vi "Text to Timestamp.vi"(8 "error in (no error)":errorcluster, 9 "initial scan location":u32, 11 "Text Timestamp":string) -> (0 "error out":errorcluster, 1 "Offset Past Timestamp":u32, 2 "Local Time Offset (NaN if unspecified)":dbl, 3 "Time Stamp":timestamp format="%^<%H:%M:%S%6u\n%Y/%m/%d>T UTC")   [LabVIEW 2024, in "JDP Timestamp.lvlib"]
doc: "Supporting RFC3339, a subset of ISO8601, plus some other formats \nRFC3339--> https://tools.ietf.org/html/rfc3339 \n Examples:\n \"2020-06-25T08:50:15.123Z\"\n \"2020-06-25T09:50:15.123+01:00\"\n\nSQLite Time Functions --> https://www.sqlite.org/lang_datefunc.html\n Examples:\n \"2020-06-25 08:50:15\" --> datetime() function\n\nAlso accepts reduced formats omitting some of the separators, or replacing them with spaces:\n \"2020 06 25 085015Z\"\n\nTo support older versions of Windows Powershell (ConvertTo-Json commandlet), also supports milliseconds since the Unix Epoch, in /Date(nnn)/ format:\n \"/Date(1608992240123)/\""
uses:
  JDP Timestamp.lvlib
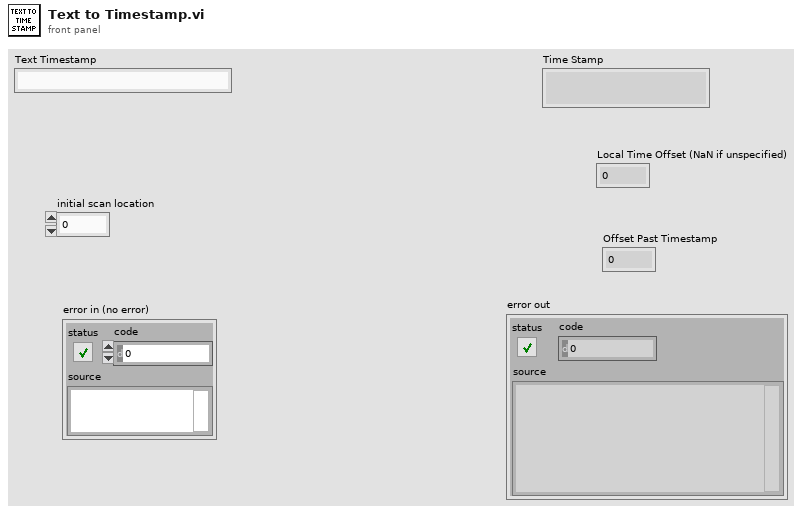
[diagram p1: front panel]
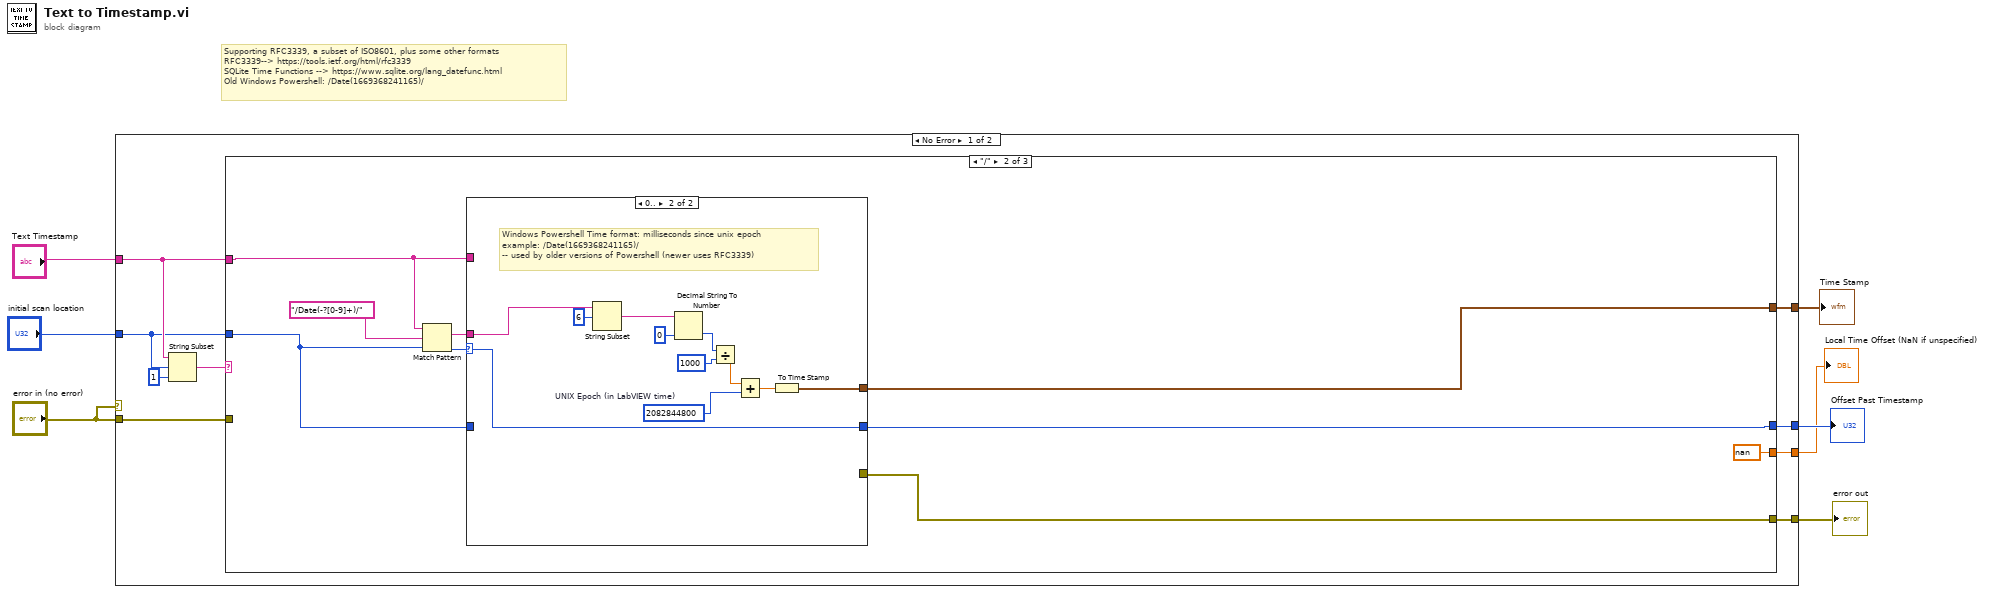
[diagram p0: block diagram]
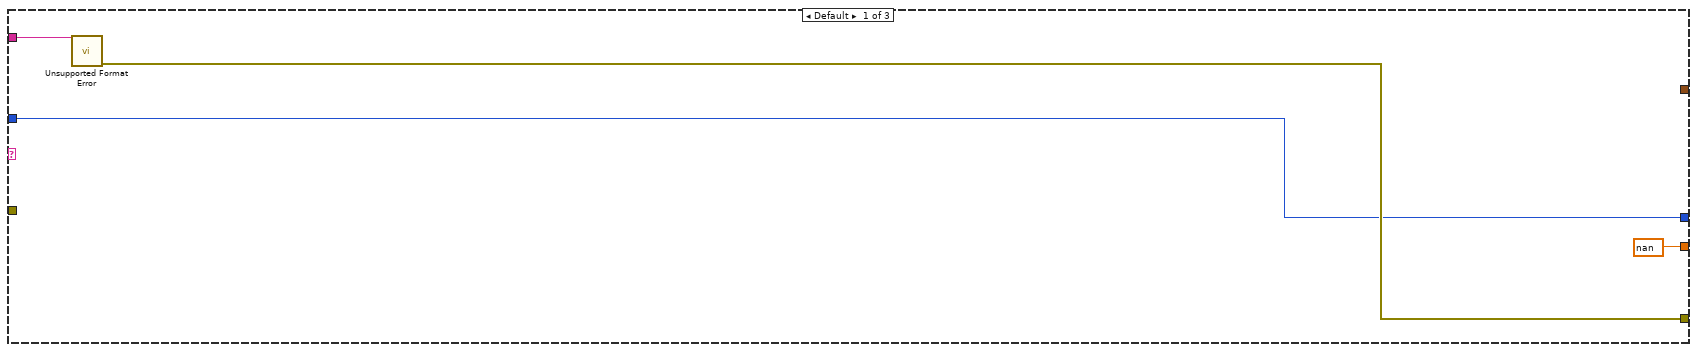
[diagram p2: hidden frame]
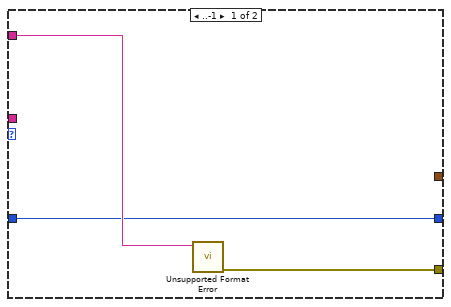
[diagram p3: hidden frame]
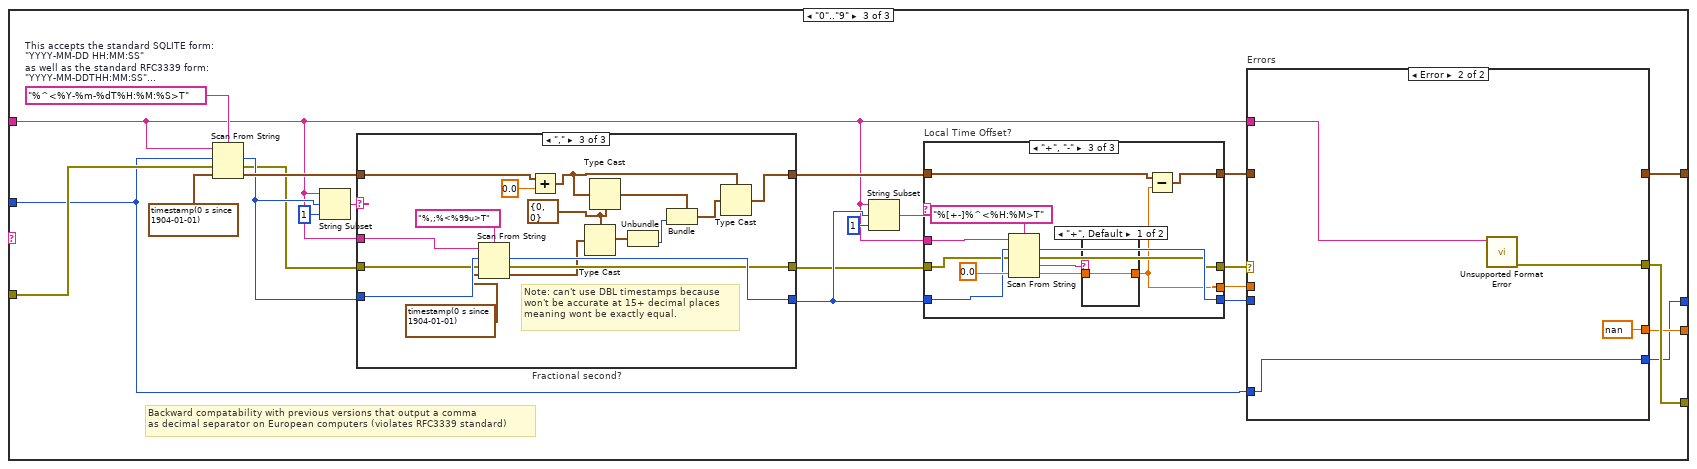
[diagram p4: hidden frame]
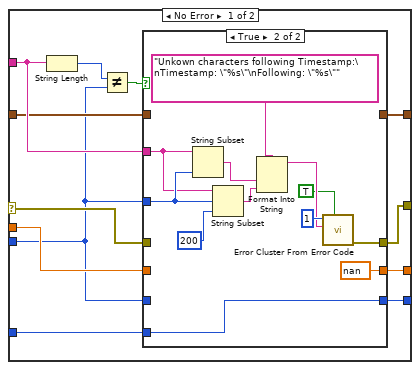
[diagram p5: hidden frame]
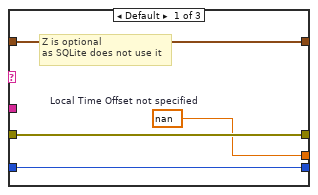
[diagram p7: hidden frame]
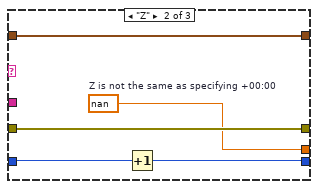
[diagram p8: hidden frame]
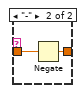
[diagram p9: hidden frame]
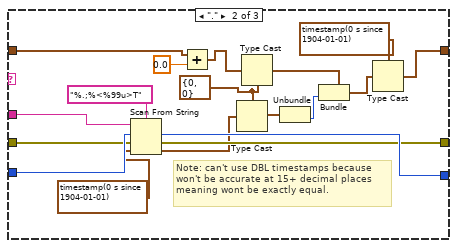
[diagram p11: hidden frame]
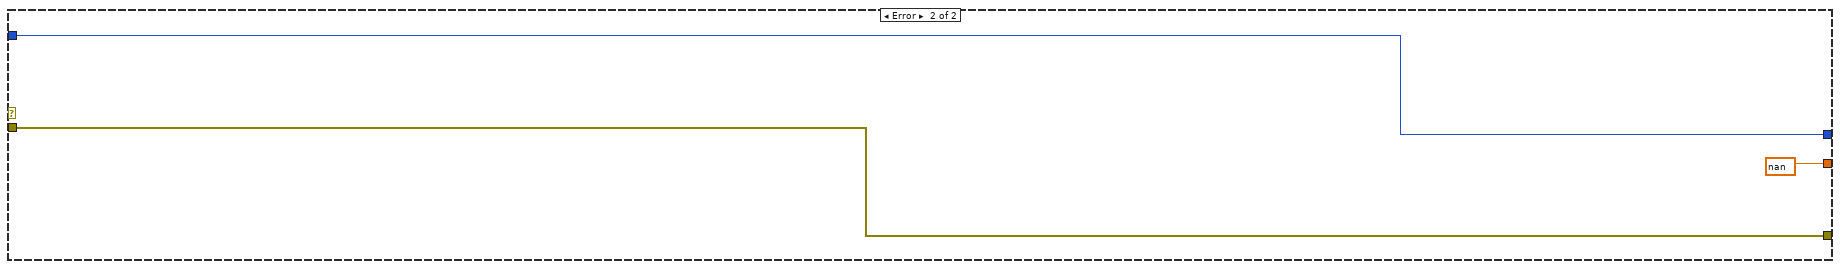
[diagram p12: hidden frame]
diagram:
  # "Supporting RFC3339, a subset of ISO8601, plus some other formats \nRFC3339--> https://tools.ietf.org/html/rfc3339\nSQLite Time Functions --> https://www.sqlite.org/lang_datefunc.html\nOld Windows Powershell: /Date(1669368241165)/"
  n1 = case shown="No Error" "error in (no error)" {
    tunnel: "Text Timestamp" -> [w11 _]
    tunnel: [w14 _] -> w6
    tunnel: [w12 w161] -> w5
    tunnel: "error in (no error)" -> [w16 w163]
    tunnel: [w15 w163] -> w4
    tunnel: [w13 nan] -> w2
    tunnel: "initial scan location" -> [w10 w161]
    frame No Error {
      n2 = String Subset(string=w11, offset (0)=w10, length (rest)=1 ("length (rest)")) -> (substring=w8:string)
      n3 = case shown="\"/\"" w8 {
        tunnel: w16 -> [_ _ w56]
        tunnel: w11 -> [w20 w26 w53]
        tunnel: [w19 w25 w50] -> w15
        tunnel: [_ w24 w48] -> w14
        tunnel: [nan nan ("Z is not the same as specifying +00:00") w46] -> w13
        tunnel: [w17 w23 w45] -> w12
        tunnel: w10 -> [w17 w21 w44]
        frame Default {
          n4 = call "Unsupported Format Error.vi"("Text Timestamp"=w20) -> ("Unsupported Format Error"=w19:errorcluster)  [unwired: 10 in]
        }
        frame "/" {
          n5 = Match Pattern(string=w26, regular expression="/Date(-?[0-9]+)/" ("format string"), offset (0)=w21) -> (match substring=w28:string, offset past match=w27:i32)  [unwired: 2 out]
          n6 = case shown="0.." w27 {
            selector: w27 -> [_ w33]
            tunnel: w28 -> [_ w43]
            tunnel: [_ w34] -> w24
            tunnel: w26 -> [w32 _]
            tunnel: [w31 _] -> w25
            tunnel: [w30 w33] -> w23
            tunnel: w21 -> [w30 _]
            frame ..-1 {
              n7 = call "Unsupported Format Error.vi"("Text Timestamp"=w32) -> ("Unsupported Format Error"=w31:errorcluster)  [unwired: 10 in]
            }
            frame 0.. {
              w36 = i64 2082844800  # UNIX Epoch (in LabVIEW time)
              # "Windows Powershell Time format: milliseconds since unix epoch\nexample: /Date(1669368241165)/\n-- used by older versions of Powershell (newer uses RFC3339)"
              n8 = String Subset(string=w43, offset (0)=6) -> (substring=w41:string)  [unwired: 1 in]
              n9 = Decimal String To Number(string=w41, default (0L)=u64 0 ("default (0 I32)")) -> (number=w39:u64)  [unwired: 1 in, 1 out]
              n10 = Divide(x=w39, y=u64 1000) -> (x/y=w37:dbl)
              n11 = Add(x=w37, y=w36) -> (x+y=w35:dbl)
              n12 = To Time Stamp(1:w35) -> (0:w34:timestamp)
            }
          }
        }
        frame "0".."9" {
          w58 = "%^<%Y-%m-%dT%H:%M:%S>T"  # This accepts the standard SQLITE form: "YYYY-MM-DD HH:MM:SS"  as well as the standard RFC3339 form: "YYYY-MM-DDTHH:MM:SS" and ISO-8601 reduced forms that don't include some/all of the -, : or T: "YYYYMMDDHHMMSS"
          # "Backward compatability with previous versions that output a comma\nas decimal separator on European computers (violates RFC3339 standard)"
          n13 = Scan From String(format string=w58, input string=w53, initial scan location=w44, error in=w56, default 1=timestamp(0 s since 1904-01-01)) -> (offset past scan=w62:u32, error out=w55:errorcluster, output 1=w63:timestamp)  [unwired: 1 out]
          n14 = String Subset(string=w53, offset (0)=w62, length (rest)=1 ("length (rest)")) -> (substring=w64:string)
          n15 = case "Fractional second?" shown="\",\"" w64 {
            tunnel: w62 -> [w124 w140 w157]
            tunnel: w53 -> [_ w143 w160]
            tunnel: w63 -> [w125 w142 w159]
            tunnel: [w125 w141 w158] -> w61
            tunnel: [w124 w139 w156] -> w57
            tunnel: w55 -> [w123 w138 w155]
            tunnel: [w123 w137 w154] -> w54
            frame Default {
            }
            frame "." {
              w132 = cluster{i64, u64} {0, 0}
              # "Note: can't use DBL timestamps because\nwon't be accurate at 15+ decimal places\nmeaning wont be exactly equal."
              n16 = Scan From String(format string="%.;%<%99u>T", input string=w143, initial scan location=w140, error in=w138, default 1=timestamp(0 s since 1904-01-01)) -> (offset past scan=w139:u32, error out=w137:errorcluster, output 1=w133:timestamp)  [unwired: 1 out]
              n17 = Add(x=w142, y=0.0) -> (x+y=w127:timestamp)
              n18 = Type Cast(type=w132, x=w133) -> (*(type *) &x=w130:cluster{i64, u64})
              n19 = Type Cast(type=w132, x=w127) -> (*(type *) &x=w131:cluster{i64, u64})
              n20 = Unbundle(w130) -> (w129:u64)  [unwired: 1 out]
              n21 = Bundle(cluster=w131, w129) -> (w128:cluster{i64, u64})  [unwired: 1 in]
              n22 = Type Cast(type=timestamp(0 s since 1904-01-01) ("x+y"), x=w128) -> (*(type *) &x=w141:timestamp)
            }
            frame "," {
              w149 = cluster{i64, u64} {0, 0}
              # "Note: can't use DBL timestamps because\nwon't be accurate at 15+ decimal places\nmeaning wont be exactly equal."
              n23 = Scan From String(format string="%,;%<%99u>T", input string=w160, initial scan location=w157, error in=w155, default 1=timestamp(0 s since 1904-01-01)) -> (offset past scan=w156:u32, error out=w154:errorcluster, output 1=w150:timestamp)  [unwired: 1 out]
              n24 = Add(x=w159, y=0.0) -> (x+y=w144:timestamp)
              n25 = Type Cast(type=w149, x=w150) -> (*(type *) &x=w147:cluster{i64, u64})
              n26 = Type Cast(type=w149, x=w144) -> (*(type *) &x=w148:cluster{i64, u64})
              n27 = Unbundle(w147) -> (w146:u64)  [unwired: 1 out]
              n28 = Bundle(cluster=w148, w146) -> (w145:cluster{i64, u64})  [unwired: 1 in]
              n29 = Type Cast(type=w144, x=w145) -> (*(type *) &x=w158:timestamp)
            }
          }
          n30 = String Subset(string=w53, offset (0)=w57, length (rest)=1 ("length (rest)")) -> (substring=w59:string)
          n31 = case "Local Time Offset?" shown="\"+\", \"-\"" w59 {
            tunnel: w57 -> [w101 w106 w114]
            tunnel: w53 -> [_ _ w118]
            tunnel: w61 -> [w102 w107 w117]
            tunnel: [w102 w107 w115] -> w49
            tunnel: [w101 w105 w113] -> w52
            tunnel: w54 -> [w100 w104 w112]
            tunnel: [w100 w104 w111] -> w51
            tunnel: [w99 w103 w109] -> w47
            frame Default {
              w99 = nan  # Local Time Offset not specified
              # "Z is optional\nas SQLite does not use it"
            }
            frame "Z" {
              w103 = nan  # Z is not the same as specifying +00:00
              n32 = Increment(x=w106) -> (x+1=w105:u32)
            }
            frame "+", "-" {
              n33 = Scan From String(format string="%[+-]%^<%H:%M>T", input string=w118, initial scan location=w114, error in=w112, default 2=0.0) -> (offset past scan=w113:u32, error out=w111:errorcluster, output 1=w108:string, output 2=w110:dbl)  [unwired: 1 in, 1 out]
              n34 = case shown="\"+\", Default" w108 {
                tunnel: w110 -> [w120 w122]
                tunnel: [w120 w121] -> w109
                frame "+", Default {
                }
                frame "-" {
                  n35 = Negate(x=w122) -> (-x=w121:dbl)
                }
              }
              n36 = Subtract(x=w117, y=w109) -> (x-y=w115:timestamp)
            }
          }
          n37 = case "Errors" shown="Error" w51 {
            selector: w51 -> [w74 _]
            tunnel: w53 -> [w76 w98]
            tunnel: w52 -> [w68 _]
            tunnel: [w77 w97] -> w50
            tunnel: w49 -> [w72 _]
            tunnel: [w73 _] -> w48
            tunnel: w47 -> [w71 _]
            tunnel: [w70 nan] -> w46
            tunnel: [w69 w95] -> w45
            tunnel: w44 -> [w67 w95]
            frame No Error {
              n38 = String Length(string=w76) -> (length=w78:i32)
              n39 = Not Equal?(x=w78, y=w68) -> (x != y?=w75:bool)
              n40 = case shown="True" w75 {
                tunnel: [w82 w88] -> w77
                tunnel: w68 -> [_ w87]
                tunnel: w76 -> [_ w86]
                tunnel: w74 -> [w82 _]
                tunnel: [w81 _] -> w73
                tunnel: w72 -> [w81 _]
                tunnel: w71 -> [w80 _]
                tunnel: [w80 nan] -> w70
                tunnel: [w79 w83] -> w69
                tunnel: w68 -> [w79 _]
                tunnel: w67 -> [_ w83]
                frame False {
                }
                frame True {
                  n41 = String Subset(string=w86, length (rest)=w87) -> (substring=w85:string)  [unwired: 1 in]
                  n42 = String Subset(string=w86, offset (0)=w87, length (rest)=200 ("length (rest)")) -> (substring=w92:string)
                  n43 = Format Into String(format string="Unkown characters following Timestamp:\nTimestamp: \"%s\"\nFollowing: \"%s\"", w85, w92) -> (resulting string=w90:string)  [unwired: 2 in, 1 out]
                  n44 = call "Error Cluster From Error Code.vi"("show call chain? (False)"=TRUE, "error message (\"\")"=w90, "error code (0)"=1) -> ("error out"=w88:errorcluster)  [unwired: 6 in]
                }
              }
            }
            frame Error {
              n45 = call "Unsupported Format Error.vi"("Text Timestamp"=w98) -> ("Unsupported Format Error"=w97:errorcluster)  [unwired: 10 in]
            }
          }
        }
      }
    }
    frame Error {
    }
  }
  "Time Stamp" <- w6
  "Offset Past Timestamp" <- w5
  "error out" <- w4
  "Local Time Offset (NaN if unspecified)" <- w2
